vi "Initialize Instrument Refs.vi"(8 "error in (no error)":errorcluster, 11 "Device Reference in":T14 format="%.0x") -> (0 "error out":errorcluster, 3 "Parameters":T1 {"Compiled"."External Channels"."Channels" format="%.0x"; "Compiled"."External Channels"."Triggers" format="%.0x"})   [LabVIEW 2019, in "Instrument Addon Engine.lvlib"]
uses:
  Instrument Addon Engine.lvlib
  Shared/Types/Linked Channel Cluster.ctl
  Shared/Instrument Addon Shared.lvlib
  Shared/Types/Command Parameters.ctl
  <vilib>/NI VeriStand/Custom Device API/Data Reference.ctl
  <vilib>/NI VeriStand/Custom Device API/Custom Device API.lvlib
  Types/Commands RT Configuration Cluster.ctl
  Shared/Types/Response Wait Type.ctl
  Shared/Types/Response Parameters.ctl
  Shared/Types/Response RT Configuration Cluster.ctl
  Shared/Types/Message Generation Type.ctl
  Shared/Types/Message Parameters.ctl
  Shared/Types/External Trigger Refs.ctl
  Shared/Types/Compiled Settings.ctl
  Shared/Constants.vi
  Protocols.lvlibp/Protocol Parent/Protocol Parent.lvclass
  Protections.lvlibp/Parent Protection/Protection.lvclass
  Shared/Types/FG Control.ctl
  Protocols.lvlibp/TCP/TCP.lvclass
  Protocols.lvlibp/UDP/UDP.lvclass
  Protocols.lvlibp/RS-xxx/RS-xxx.lvclass
  <vilib>/NI VeriStand/Custom Device Tools/Custom Device Utility Library/Custom Device Utility Library.lvlib
  Shared/Types/Command Channel Index.ctl
  Shared/Types/Command Channel Indeces.ctl
  <vilib>/NI VeriStand/Custom Device Tools/Custom Device Utility Library/NI VeriStand - Search for All Items by GUID.vi
  <vilib>/NI VeriStand/Custom Device API/Get Item Property (Variant).vi
  Protocols.lvlibp/VISA/VISA.lvclass
  C:/Addons/Instrument-Custom-Device/Source/Protocols.lvlibp/Protocol Parent/Protocol Parent.lvclass
  <vilib>/NI VeriStand/Custom Device API/Custom Device Item Ref.ctl
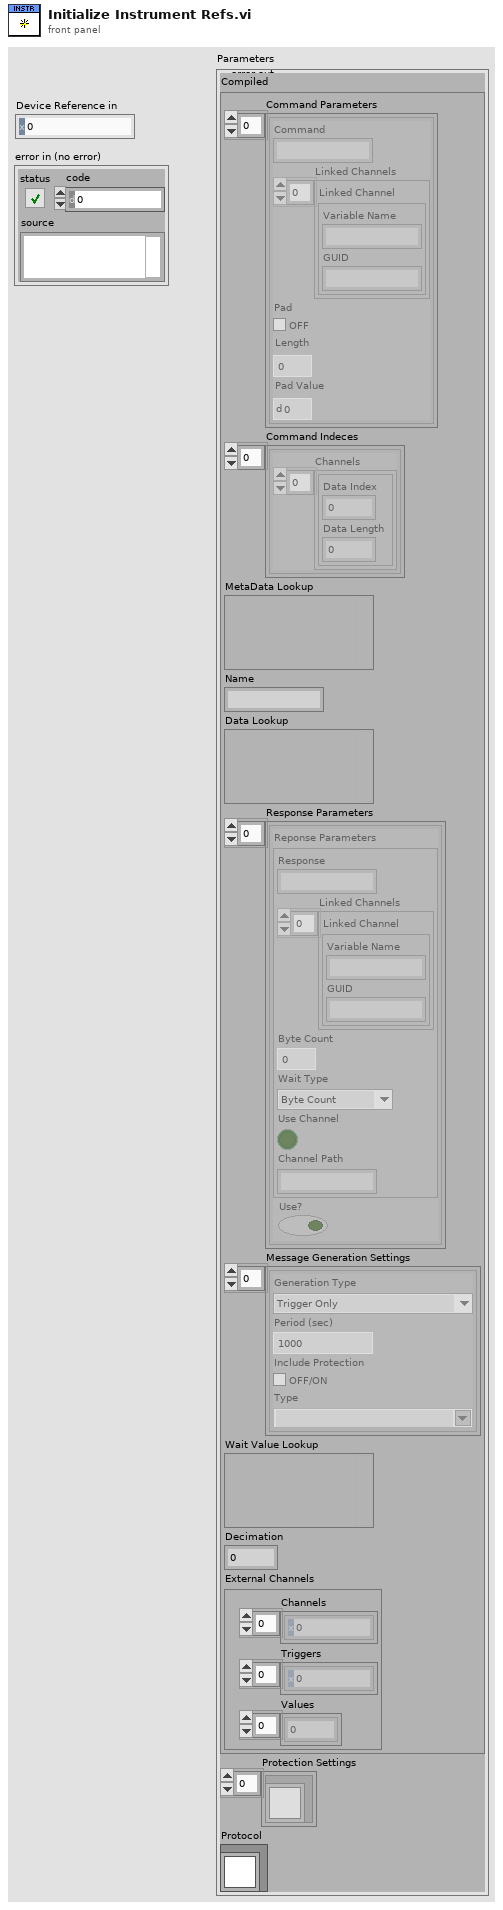
[diagram p1: front panel]
types:
  T1 = typedef "Instrument Addon Engine.lvlib/Commands RT Configuration Cluster.ctl" = cluster{"Compiled":T2, "Protection Settings":refnum<class "Protection.lvclass">[], "Protocol":refnum<class "Protocol Parent.lvclass">}
  T2 = typedef "Instrument Addon Shared.lvlib/Compiled Settings.ctl" = cluster{"Command Parameters":T3[], "Command Indeces":T5[], "MetaData Lookup":variant, "Name":string, "Data Lookup":variant, "Response Parameters":T7[], "Message Generation Settings":T10[], "Wait Value Lookup":variant, "Decimation":u32, "External Channels":T12}
  T3 = typedef "Instrument Addon Shared.lvlib/Command Parameters.ctl" = cluster{"Command":string, "Linked Channels":T4[], "Pad":bool, "Length":u32, "Pad Value":u8}
  T4 = typedef "Instrument Addon Shared.lvlib/Linked Channel Cluster.ctl" = cluster{"Variable Name":string, "GUID":string}
  T5 = typedef "Instrument Addon Shared.lvlib/Command Channel Indeces.ctl" = cluster{"Channels":T6[]}
  T6 = typedef "Instrument Addon Shared.lvlib/Command Channel Index.ctl" = cluster{"Data Index":i32, "Data Length":i32}
  T7 = typedef "Instrument Addon Shared.lvlib/Response RT Configuration Cluster.ctl" = cluster{"Reponse Parameters":T8, "Use?":bool}
  T8 = typedef "Instrument Addon Shared.lvlib/Response Parameters.ctl" = cluster{"Response":string, "Linked Channels":T4[], "Type Value":dbl, "Wait Type":T9, "Use Channel":bool, "Channel Path":string}
  T9 = typedef "Instrument Addon Shared.lvlib/Response Wait Type.ctl" = enum16{"Byte Count", "Wait sec"}
  T10 = typedef "Instrument Addon Shared.lvlib/Message Parameters.ctl" = cluster{"Generation Type":T11, "Period":dbl, "Include Protection":bool, "Type":string}
  T11 = typedef "Instrument Addon Shared.lvlib/Message Generation Type.ctl" = enum16{"Trigger Only", "Periodic & Trigger", "Value Change & Trigger"}
  T12 = typedef "Instrument Addon Shared.lvlib/External Trigger Refs.ctl" = cluster{"Channels":T13[], "Triggers":T13[], "Values":dbl[]}
  T13 = typedef "Custom Device API.lvlib/Data Reference.ctl" = i32
  T14 = typedef "Custom Device API.lvlib/Custom Device Item Ref.ctl" = u64
  T15 = typedef "Instrument Addon Shared.lvlib/FG Control.ctl" = enum16{"Get", "Set"}
  T16 = typedef "Protocols.lvlibp/Protocol Parent.lvclass/Base Protocol Type.ctl" = enum16{"RS-XXX", "VISA", "TCPIP", "UDP"}
  T17 = typedef "Instrument Addon Shared.lvlib/VISA Settings.ctl" = cluster{"VISA Resource":string, "Enable Termination Character":bool, "Termination Character":u8, "Timeout":u32, "Append Write Termination Character":bool}
  T18 = typedef "Instrument Addon Shared.lvlib/TCPIP Settings.ctl" = cluster{"IP Address":string, "Port":u16}
  T19 = typedef "Instrument Addon Shared.lvlib/UDP Settings.ctl" = cluster{"Local IP Address":string, "Local Port":u16, "Target IP Address":string, "Target Port":u16}
  T20 = typedef "Instrument Addon Shared.lvlib/RSXXX Port Settings.ctl" = cluster{"Port":string, "Baud Rate":u32, "Data Bits":u16, "Parity":enum16{"None", "Odd", "Even", "Mark", "Space"}, "Stop Bits":u16, "Flow Control":u16, "XON":enum16{"NUL", "SOH", "STX", "ETX", "EOT", "ENQ", "ACK", "BEL", "BS", "HT", "LF", "VT", "FF", "CR", "SO", "SI", "DLE", "DC1", "DC2", "DC3", "DC4", "NAK", "SYN", "ETB", "CAN", "EM", "SUB", "ESC", "FS", "GS", "RS", "US", "SP", "!", "\"", "#", "$", "%", "&", "'", "(", ")", "*", "+", ",", "- (-)", ".", "/", "0", "1", "2", "3", "4", "5", "6", "7", "8", "9", ":", ";", "<", "=", ">", "?", "@", "A", "B", "C", "D", "E", "F", "G", "H", "I", "J", "K", "L", "M", "N", "O", "P", "Q", "R", "S", "T", "U", "V", "W", "X", "Y", "Z", "[", "\\", "]", "^", "_", "`", "a", "b", "c", "d", "e", "f", "g", "h", "i", "j", "k", "l", "m", "n", "o", "p", "q", "r", "s", "t", "u", "v", "w", "x", "y", "z", "{", "|", "}", "~"}, "XOFF":enum16{"NUL", "SOH", "STX", "ETX", "EOT", "ENQ", "ACK", "BEL", "BS", "HT", "LF", "VT", "FF", "CR", "SO", "SI", "DLE", "DC1", "DC2", "DC3", "DC4", "NAK", "SYN", "ETB", "CAN", "EM", "SUB", "ESC", "FS", "GS", "RS", "US", "SP", "!", "\"", "#", "$", "%", "&", "'", "(", ")", "*", "+", ",", "- (-)", ".", "/", "0", "1", "2", "3", "4", "5", "6", "7", "8", "9", ":", ";", "<", "=", ">", "?", "@", "A", "B", "C", "D", "E", "F", "G", "H", "I", "J", "K", "L", "M", "N", "O", "P", "Q", "R", "S", "T", "U", "V", "W", "X", "Y", "Z", "[", "\\", "]", "^", "_", "`", "a", "b", "c", "d", "e", "f", "g", "h", "i", "j", "k", "l", "m", "n", "o", "p", "q", "r", "s", "t", "u", "v", "w", "x", "y", "z", "{", "|", "}", "~"}, "End Read on Termination Character":bool, "End Write on Termination Character":bool, "Termination Character":u8}
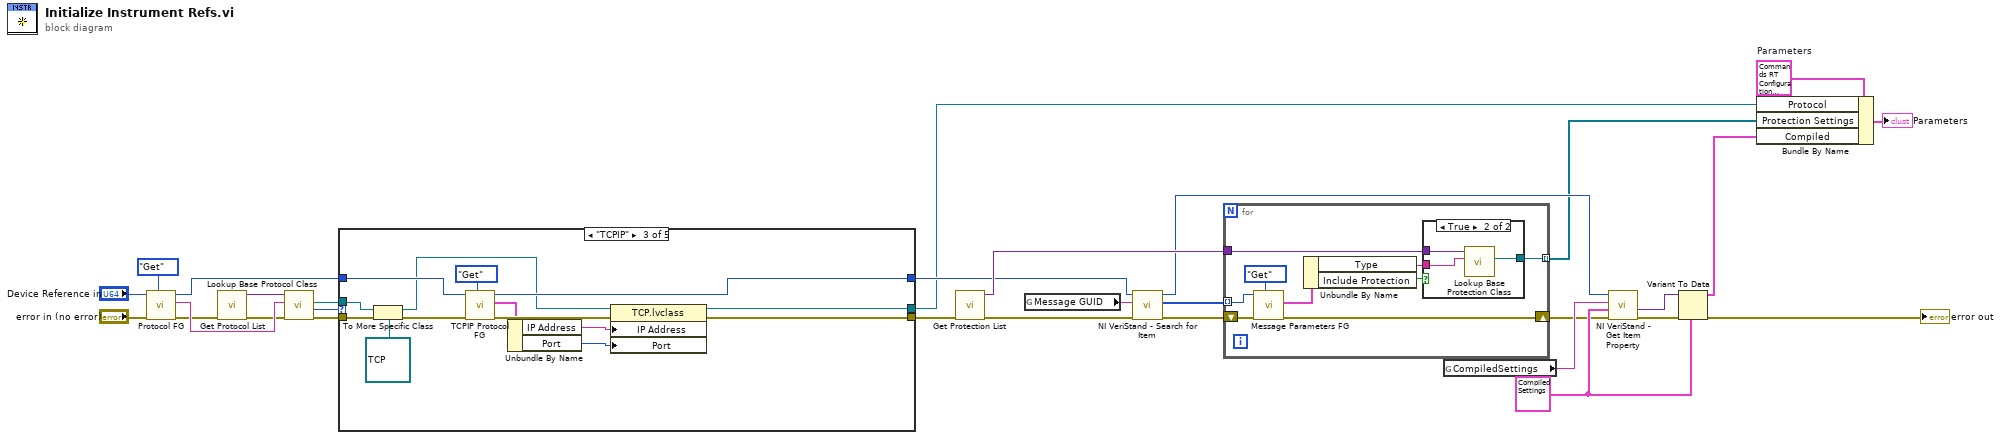
[diagram p0: block diagram]
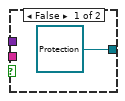
[diagram p2: hidden frame]
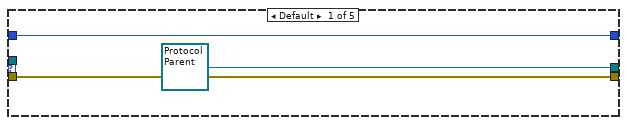
[diagram p3: hidden frame]
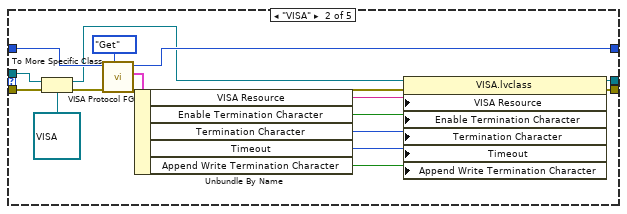
[diagram p4: hidden frame]
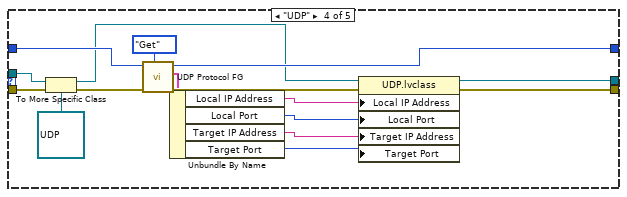
[diagram p5: hidden frame]
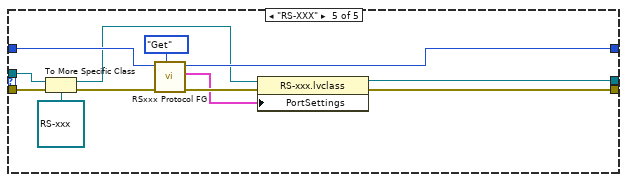
[diagram p6: hidden frame]
diagram:
  w25 = T2 {"Command Parameters"=[], "Command Indeces"=[], "MetaData Lookup"=variant, "Name"="", "Data Lookup"=variant, "Response Parameters"=[], "Message Generation Settings"=[], "Wait Value Lookup"=variant, "Decimation"=0, "External Channels"={"Channels"=[], "Triggers"=[], "Values"=[]}} ("Parameters")
  w30 = T1 {"Compiled"={"Command Parameters"=[], "Command Indeces"=[], "MetaData Lookup"=variant, "Name"="", "Data Lookup"=variant, "Response Parameters"=[], "Message Generation Settings"=[], "Wait Value Lookup"=variant, "Decimation"=0, "External Channels"={"Channels"=[], "Triggers"=[], "Values"=[]}}, "Protection Settings"=[], "Protocol"=refnum}  # Parameters
  n1 = call "Protocol FG.vi"("Action"=FG_Control."Get", "error in (no error)"="error in (no error)", "Device Item Ref in"="Device Reference in") -> ("error out"=w17:errorcluster, "Protocol out"=w23:string, "Item Ref out"=w16:T14)  [unwired: 6 in]
  n2 = call "Get Protocol List.vi"("error in (no error)"=w17) -> ("error out"=w19:errorcluster, "Class Lookup"=w18:variant)  [unwired: 9 in]
  n3 = call "Lookup Base Protocol Class.vi"("error in (no error)"=w19, "Protocol in"=w23, "Class Lookup"=w18) -> ("error out"=w22:errorcluster, "Protocol out"=w21:T16, "Protocol Parent out"=w20:refnum<class "Protocol Parent.lvclass">)  [unwired: 5 in, 1 out]
  n4 = case shown="\"TCPIP\"" w21 {
    tunnel: w16 -> [w32 w48 w61 w77 w91]
    tunnel: w22 -> [w33 w38 w54 w70 w84]
    tunnel: [w33 w50 w64 w80 w88] -> w4
    tunnel: [w32 w47 w60 w76 w90] -> w6
    tunnel: [refnum<class "Protocol Parent.lvclass"> refnum ("Protocols.lvlibp:Protocol Parent.lvclass") w49 w63 w79 w87] -> w2
    tunnel: w20 -> [_ w42 w55 w71 w85]
    frame Default {
    }
    frame "VISA" {
      n5 = To More Specific Class(target class=refnum<class "VISA.lvclass"> refnum ("Protocols.lvlibp:VISA.lvclass"), reference=w42, error in=w38) -> (specific class reference=w41:refnum<class "VISA.lvclass">, error out=w40:errorcluster)
      n6 = call "VISA Protocol FG.vi"("Action"=FG_Control."Get", "error in (no error)"=w40, "Device Item Ref in"=w48) -> ("error out"=w39:errorcluster, "VISA Config"=w45:T17, "Item Ref out"=w47:T14)  [unwired: 6 in]
      n7 = Unbundle By Name(w45) -> ("VISA Resource"=w44:string, "Enable Termination Character"=w36:bool, "Termination Character"=w37:u8, "Timeout"=w34:u32, "Append Write Termination Character"=w35:bool)
      n8 = property class="VISA.lvclass"(reference=w41, error in=w39, "VISA Resource"=w44, "Enable Termination Character"=w36, "Termination Character"=w37, "Timeout"=w34, "Append Write Termination Character"=w35) -> (reference out=w49:refnum<class "VISA.lvclass">, error out=w50:errorcluster)
    }
    frame "TCPIP" {
      n9 = To More Specific Class(target class=refnum<class "TCP.lvclass"> refnum ("Protocols.lvlibp:TCP.lvclass"), reference=w55, error in=w54) -> (specific class reference=w52:refnum<class "TCP.lvclass">, error out=w53:errorcluster)
      n10 = call "TCPIP Protocol FG.vi"("Action"=FG_Control."Get", "error in (no error)"=w53, "Device Item Ref in"=w61) -> ("error out"=w62:errorcluster, "TCP/IP Config"=w58:T18, "Item Ref out"=w60:T14)  [unwired: 6 in]
      n11 = Unbundle By Name(w58) -> ("IP Address"=w57:string, "Port"=w56:u16)
      n12 = property class="TCP.lvclass"(reference=w52, error in=w62, "IP Address"=w57, "Port"=w56) -> (reference out=w63:refnum<class "TCP.lvclass">, error out=w64:errorcluster)
    }
    frame "UDP" {
      n13 = To More Specific Class(target class=refnum<class "UDP.lvclass"> refnum ("Protocols.lvlibp:UDP.lvclass"), reference=w71, error in=w70) -> (specific class reference=w65:refnum<class "UDP.lvclass">, error out=w69:errorcluster)
      n14 = call "UDP Protocol FG.vi"("Action"=FG_Control."Get", "error in (no error)"=w69, "Device Item Ref in"=w77) -> ("error out"=w78:errorcluster, "UDP Config"=w74:T19, "Item Ref out"=w76:T14)  [unwired: 6 in]
      n15 = Unbundle By Name(w74) -> ("Local IP Address"=w73:string, "Local Port"=w72:u16, "Target IP Address"=w67:string, "Target Port"=w66:u16)
      n16 = property class="UDP.lvclass"(reference=w65, error in=w78, "Local IP Address"=w73, "Local Port"=w72, "Target IP Address"=w67, "Target Port"=w66) -> (reference out=w79:refnum<class "UDP.lvclass">, error out=w80:errorcluster)
    }
    frame "RS-XXX" {
      n17 = To More Specific Class(target class=refnum<class "RS-xxx.lvclass"> refnum ("Protocols.lvlibp:RS-xxx.lvclass"), reference=w85, error in=w84) -> (specific class reference=w81:refnum<class "RS-xxx.lvclass">, error out=w83:errorcluster)
      n18 = call "RSxxx Protocol FG.vi"("Action"=FG_Control."Get", "error in (no error)"=w83, "Device Item Ref in"=w91) -> ("error out"=w89:errorcluster, "Serial Config"=w86:T20, "Item Ref out"=w90:T14)  [unwired: 6 in]
      n19 = property class="RS-xxx.lvclass"(reference=w81, error in=w89, "PortSettings"=w86) -> (reference out=w87:refnum<class "RS-xxx.lvclass">, error out=w88:errorcluster)
    }
  }
  n20 = call "Get Protection List.vi"("error in (no error)"=w4) -> ("error out"=w9:errorcluster, "Class Lookup"=w8:variant)  [unwired: 9 in]
  n21 = global read "Constants.vi" "Message GUID"() -> (w12:string)
  n22 = call-poly <vilib>:"NI VeriStand - Search for Item.vi"("error in"=w9, "Item GUID"=w12, "Section Ref in"=w6) -> ("error out"=w10:errorcluster, "Item Refs"=w11:T14[], "Section Ref out"=w7:T14)  [unwired: 5 in, 1 out]
  n23 = for {
    tunnel: w11 -> [w100] mode=indexing
    shift-right: [w93] -> w5
    shift-left: w10 -> [w101]
    tunnel: w8 -> [w97]
    tunnel: [w96] -> w3 mode=indexing
    n24 = call "Message Parameters FG.vi"("Action"=FG_Control."Get", "error in (no error)"=w101, "Item Ref in"=w100) -> ("error out"=w93:errorcluster, "Message Settings out"=w98:T10)  [unwired: 6 in, 1 out]
    n25 = Unbundle By Name(w98) -> ("Type"=w95:string, "Include Protection"=w94:bool)
    n26 = case shown="True" w94 {
      tunnel: w97 -> [_ w105]
      tunnel: w95 -> [_ w104]
      tunnel: [refnum<class "Protection.lvclass"> refnum ("Protection.lvclass") w103] -> w96
      frame False {
      }
      frame True {
        n27 = call "Lookup Base Protection Class.vi"("Protection in"=w104, "Class Lookup"=w105) -> ("Protection.lvclass"=w103:refnum<class "Protection.lvclass">)  [unwired: 7 in, 2 out]
      }
    }
  }
  n28 = global read "Constants.vi" "CompiledSettings"() -> (w28:string)
  n29 = call-poly <vilib>:"NI VeriStand - Get Item Property.vi"("error in (no error)"=w5, "Default Value"=w25, "Property Name"=w28, "Item Ref in"=w7) -> ("error out"=w27:errorcluster, "Value"=w26:variant)  [unwired: 4 in, 2 out]
  n30 = Variant To Data(error in=w27, type=w25, Variant=w26) -> (data=w24:T2, error out=→"error out":errorcluster)
  n31 = Bundle By Name(cluster=w30, "Protocol"=w2, "Protection Settings"=w3, "Compiled"=w24) -> (→"Parameters":T1)
